vi "Process.vi"(8 "error in":errorcluster, 11 "Qbus in":refnum<class "Qbus.lvclass">) -> (0 "error out":errorcluster)   [LabVIEW 2021, in "DigitalAudioGenerationProcess.lvlib"]
uses:
  DigitalAudioGenerationProcess.lvlib
  <vilib>/addons/Qbus/Qbus.lvclass
  controls/state.ctl
  controls/generation status.ctl
  <vilib>/PDM Acquisition Toolkit/host/Classes/Tasks/PCM Output/Controls/PCM Output Task DVR.ctl
  <vilib>/PDM Acquisition Toolkit/host/Classes/Tasks/PCM Output/PCM Output Task.lvclass
  controls/digital generation settings.ctl
  controls/digital protocol settings.ctl
  <vilib>/PDM Acquisition Toolkit/host/Classes/Session/Controls/Logic Levels.ctl
  <vilib>/PDM Acquisition Toolkit/shared/controls/PCM Data Format Configuration.ctl
  <vilib>/PDM Acquisition Toolkit/shared/controls/Digital Edge.ctl
  <vilib>/PDM Acquisition Toolkit/shared/controls/PCM Bit Endianness.ctl
  <vilib>/PDM Acquisition Toolkit/shared/controls/PCM Data Justification.ctl
  <vilib>/PDM Acquisition Toolkit/shared/controls/clock mode.ctl
  <vilib>/PDM Acquisition Toolkit/shared/controls/PCM Frame Sync Control.ctl
  <vilib>/PDM Acquisition Toolkit/host/Classes/Tasks/I2S Output/Control/SignalProperties.ctl
  <vilib>/PDM Acquisition Toolkit/host/Classes/Channels/I2S Ouput/Controls/GenerationChannelProperties.ctl
  controls/update signal settings.ctl
  <vilib>/PDM Acquisition Toolkit/host/Classes/Session/DecoderSession.lvclass
  <vilib>/PDM Acquisition Toolkit/shared/PDM Shared.lvlib
  controls/AudioGenTypeDefs.lvlib
  <vilib>/PDM Acquisition Toolkit/host/Classes/Channels/I2S Ouput/I2S Output Channel.lvclass
  <vilib>/PDM Acquisition Toolkit/host/Classes/Tasks/I2S Output/I2S Output Task.lvclass
  shared/logger process/EventLoggerProcess.lvlib
  subVIs/utility/AudioGenUtility.lvlib
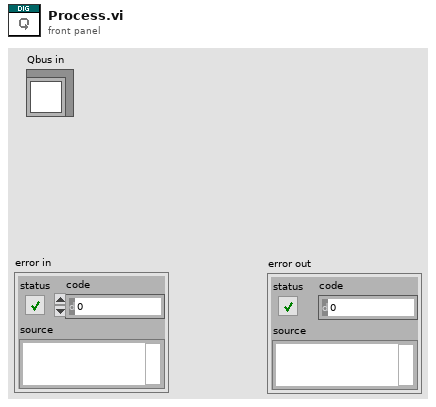
[diagram p1: front panel]
types:
  T1 = typedef "DigitalAudioGenerationProcess.lvlib/state.ctl" = cluster{"status":T2, "data task":T3, "master clock task":T3}
  T2 = typedef "AudioGenTypeDefs.lvlib/generation status.ctl" = enum16{"Idle", "Committed", "Active"}
  T3 = typedef "PDM Acquisition Class Library.lvlib/PCM Output Task.lvclass/PCM Output Task DVR.ctl" = refnum<data-value>
  T4 = typedef "AudioGenTypeDefs.lvlib/digital generation settings.ctl" = cluster{"data channel list":string, "master clock channel list":string, "digital protocol settings":T5, "signal parameters":T13}
  T5 = typedef "AudioGenTypeDefs.lvlib/digital protocol settings.ctl" = cluster{"logic level":T6, "PCM Data Configuration":T7, "bit clock rate":sgl, "master clock rate":sgl, "clock mode":T11, "Frame Sync Clock Control":T12}
  T6 = typedef "PDM Acquisition Class Library.lvlib/DecoderSession.lvclass/Logic Levels.ctl" = enum16{"3.3 V", "1.8 V", "1.2 V"}
  T7 = typedef "PDM Shared.lvlib/PCM Data Format Configuration.ctl" = cluster{"Frame Sync Edge for Channel 0":T8, "Channel Count Per Frame":u8, "Channel Length":u16, "Bit Depth":u8, "Channel 0 Offset":u16, "Endianness":T9, "Data Justification":T10}
  T8 = typedef "PDM Shared.lvlib/Digital Edge.ctl" = enum8{"Rising", "Falling"}
  T9 = typedef "PDM Shared.lvlib/PCM Bit Endianness.ctl" = enum16{"MSB First", "LSB First"}
  T10 = typedef "PDM Shared.lvlib/PCM Data Justification.ctl" = enum16{"Left Justified", "Right Justified"}
  T11 = typedef "PDM Shared.lvlib/clock mode.ctl" = enum16{"divided clock", "DDS"}
  T12 = typedef "PDM Shared.lvlib/PCM Frame Sync Control.ctl" = cluster{"Frame Length":u16, "Frame Sync Pulse Width":u16, "Bit Clock Edge  Sync":T8}
  T13 = typedef "PDM Acquisition Class Library.lvlib/I2S Output Task.lvclass/SignalProperties.ctl" = cluster{"cyclic signal":dbl[], "channel parameters":T14[]}
  T14 = typedef "PDM Acquisition Class Library.lvlib/I2S Output Channel.lvclass/GenerationChannelProperties.ctl" = cluster{"cyclic period":dbl, "cyclic phase offset":dbl, "gain":dbl}
  T15 = typedef "AudioGenTypeDefs.lvlib/update signal settings.ctl" = cluster{"frequency":dbl, "gain":dbl}
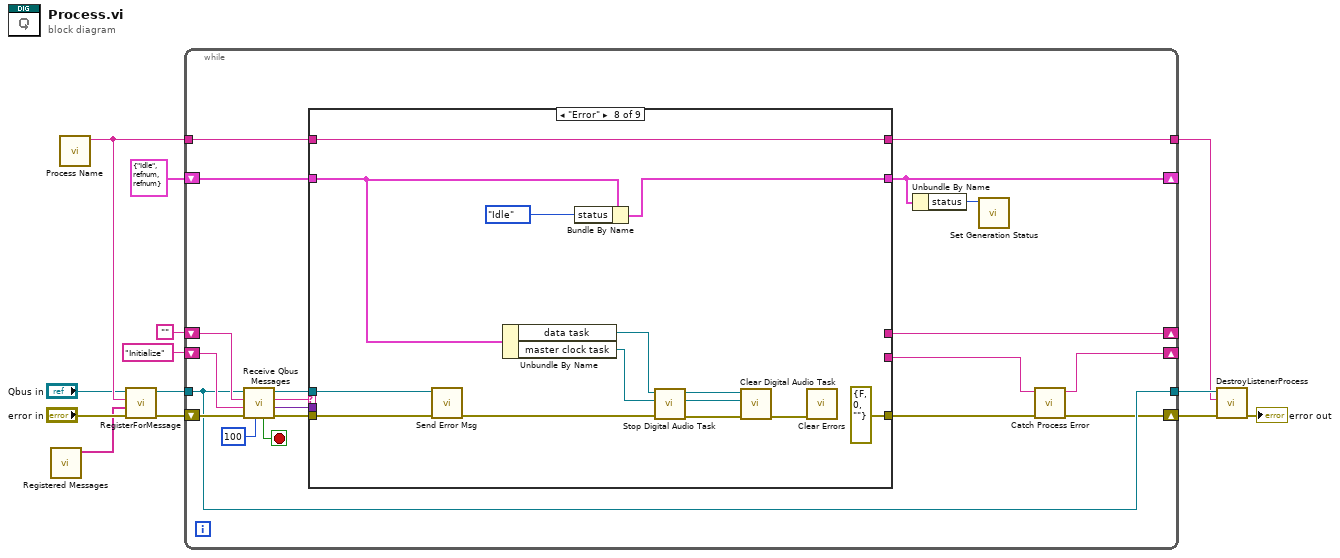
[diagram p0: block diagram]
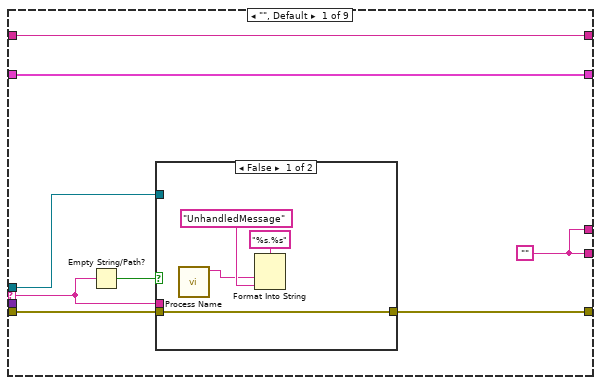
[diagram p2: hidden frame]
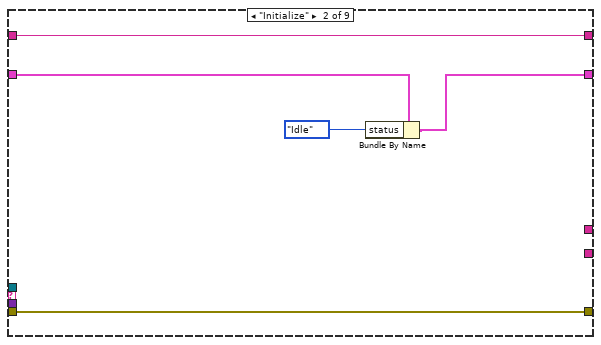
[diagram p4: hidden frame]
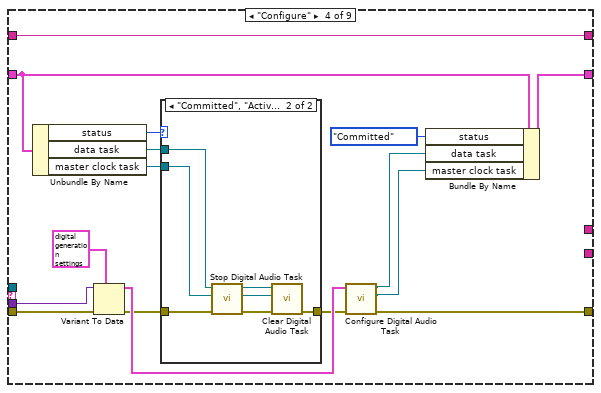
[diagram p6: hidden frame]
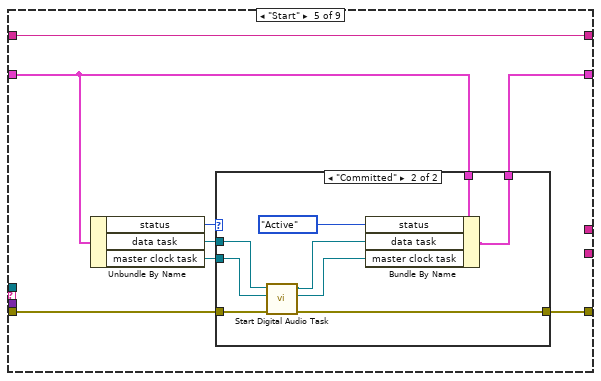
[diagram p8: hidden frame]
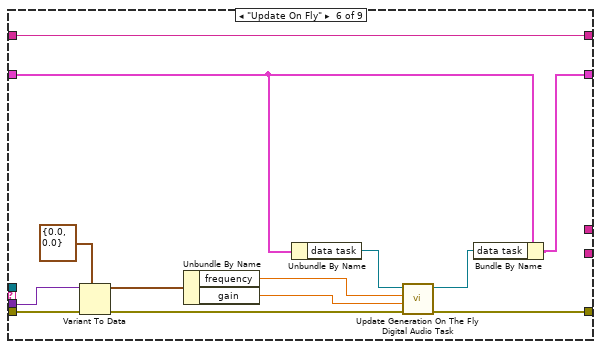
[diagram p10: hidden frame]
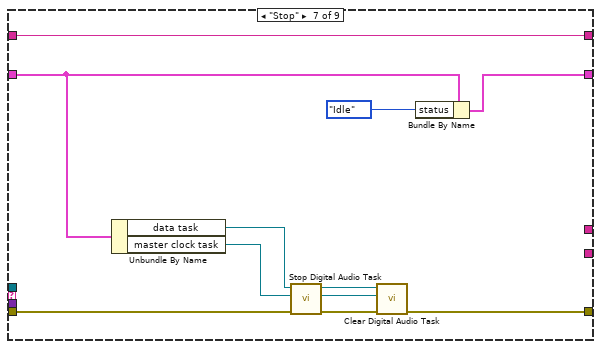
[diagram p11: hidden frame]
diagram:
  n1 = call "Registered Messages.vi"() -> ("registered messages"=w6:string[])  [unwired: 11 in]
  n2 = call "Process Name.vi"() -> ("process name"=w9:string)  [unwired: 11 in]
  n3 = call <vilib>:"RegisterForMessage.vi"("error in (no error)"="error in", "message names"=w6, "process name"=w9, "Qbus in"="Qbus in") -> ("error in (no error)"=w12:errorcluster, "Qbus out"=w13:refnum<class "Qbus.lvclass">)  [unwired: 6 in]
  n4 = while {
    shift-right: [w23] -> _
    shift-left: "" -> [w32]
    tunnel: w13 -> [w18]
    tunnel: w9 -> [w22]
    tunnel: [w18] -> w4
    tunnel: [w24] -> w2
    shift-right: [w14] -> _
    shift-left: "Initialize" -> [w28]
    shift-right: [w17] -> w5
    shift-left: w12 -> [w27]
    shift-right: [w19] -> _
    shift-left: T1 {"status"=enum."Idle", "data task"=refnum, "master clock task"=refnum} ("state") -> [w21]
    stop <- w33 stop-if-true
    n5 = call "Receive Qbus Messages.vi"("timeout(ms)"=100 ("milliseconds to wait"), "error in (no error)"=w27, "priority action"=w28, "default action"=w32, "Qbus in"=w18) -> ("error out"=w31:errorcluster, "message value"=w29:variant, "action"=w26:string, "Qbus out"=w30:refnum<class "Qbus.lvclass">, "exit"=w33:bool)  [unwired: 2 in]
    n6 = case shown="\"Error\"" w26 {
      selector: w26 -> [w38 _ _ _ _ _ _ _ _]
      tunnel: w31 -> [w40 w51 w54 w69 w85 w104 w117 w124 w138]
      tunnel: w30 -> [w36 _ _ _ _ _ _ w125 _]
      tunnel: [w39 w51 w54 w66 w80 w109 w111 errorcluster {"status"=FALSE, "code"=0, "source"=""} ("error out") w138] -> w16
      tunnel: w29 -> [_ _ _ w68 _ w103 _ _ _]
      tunnel: [w41 w50 w53 w70 w86 w110 w121 w135 w137] -> w24
      tunnel: w22 -> [w41 w50 w53 w70 w86 w110 w121 w135 w137]
      tunnel: [w35 _ _ _ _ _ _ _ _] -> w15
      tunnel: [w35 _ _ _ _ _ _ _ _] -> w23
      tunnel: w21 -> [w34 w49 w52 w60 w82 w106 w119 w133 w136]
      tunnel: [w34 w48 w52 w64 w81 w105 w118 w132 w136] -> w19
      frame "", Default {
        w35 = ""
        n7 = Empty String/Path?(string/path=w38) -> (empty?=w37:bool)
        n8 = case shown="False" w37 {
          tunnel: [w42 w46] -> w39
          tunnel: w40 -> [w42 w46]
          tunnel: w38 -> [_ _]
          tunnel: w36 -> [_ _]
          frame False {
            n9 = call "Process Name.vi"() -> ("process name"=w43:string)  [unwired: 11 in]
            n10 = Format Into String(format string="%s.%s", w43, "UnhandledMessage" ("ProcessName")) -> ()  [unwired: 2 in, 2 out]
          }
          frame True {
          }
        }
      }
      frame "Initialize" {
        n11 = Bundle By Name(cluster=w49, "status"=generation_status."Idle") -> (w48:T1)
      }
      frame "DetectHW" {
      }
      frame "Configure" {
        n12 = Unbundle By Name(w60) -> ("status"=w59:T2, "data task"=w58:T3, "master clock task"=w57:T3)
        n13 = Variant To Data(error in=w69, type=T4 {"data channel list"="", "master clock channel list"="", "digital protocol settings"={"logic level"=enum."3.3 V", "PCM Data Configuration"={"Frame Sync Edge for Channel 0"=enum."Falling", "Channel Count Per Frame"=2, "Channel Length"=32, "Bit Depth"=24, "Channel 0 Offset"=1, "Endianness"=enum."MSB First", "Data Justification"=enum."Left Justified"}, "bit clock rate"=3025000.0, "master clock rate"=3025000.0, "clock mode"=enum."divided clock", "Frame Sync Clock Control"={"Frame Length"=64, "Frame Sync Pulse Width"=32, "Bit Clock Edge  Sync"=enum."Falling"}}, "signal parameters"={"cyclic signal"=[], "channel parameters"=[]}} ("digital generation"), Variant=w68) -> (data=w65:T4, error out=w56:errorcluster)
        n14 = case shown="\"Committed\", \"Active\"" w59 {
          tunnel: w58 -> [_ w73]
          tunnel: w57 -> [_ w72]
          tunnel: w56 -> [w71 w75]
          tunnel: [w71 w74] -> w55
          frame "Idle", Default {
          }
          frame "Committed", "Active" {
            n15 = call "Stop Digital Audio Task.vi"("error in (no error)"=w75, "master clock task"=w72, "data task"=w73) -> ("error out"=w76:errorcluster, "master clock task"=w78:T3, "data task"=w77:T3)  [unwired: 6 in]
            n16 = call "Clear Digital Audio Task.vi"("error in (no error)"=w76, "master clock task"=w78, "data task"=w77) -> ("error out"=w74:errorcluster)  [unwired: 8 in]
          }
        }
        n17 = call "Configure Digital Audio Task.vi"("error in (no error)"=w55, "digital generation"=w65) -> ("error out"=w66:errorcluster, "master clock task"=w61:T3, "data task"=w62:T3)  [unwired: 7 in]
        n18 = Bundle By Name(cluster=w60, "status"=generation_status."Committed", "data task"=w62, "master clock task"=w61) -> (w64:T1)
      }
      frame "Start" {
        n19 = Unbundle By Name(w82) -> ("status"=w79:T2, "data task"=w84:T3, "master clock task"=w83:T3)
        n20 = case shown="\"Committed\"" w79 {
          tunnel: w85 -> [w88 w97]
          tunnel: w84 -> [_ w96]
          tunnel: w83 -> [_ w95]
          tunnel: w82 -> [w87 w92]
          tunnel: [w87 w91] -> w81
          tunnel: [w88 w90] -> w80
          frame "Idle", Default {
            # "not ready to start; commit first"
          }
          frame "Committed" {
            n21 = call "Start Digital Audio Task.vi"("error in (no error)"=w97, "master clock task"=w95, "data task"=w96) -> ("error out"=w90:errorcluster, "master clock task"=w93:T3, "data task"=w94:T3)  [unwired: 6 in]
            n22 = Bundle By Name(cluster=w92, "status"=generation_status."Active", "data task"=w94, "master clock task"=w93) -> (w91:T1)
          }
        }
      }
      frame "Update On Fly" {
        n23 = Variant To Data(error in=w104, type=T15 {"frequency"=0.0, "gain"=0.0} ("signal update setting"), Variant=w103) -> (data=w101:T15, error out=w100:errorcluster)
        n24 = Unbundle By Name(w101) -> ("frequency"=w99:dbl, "gain"=w98:dbl)
        n25 = Unbundle By Name(w106) -> ("data task"=w107:T3)
        n26 = call "Update Generation On The Fly Digital Audio Task.vi"("error in (no error)"=w100, "gain"=w98, "frequency"=w99, "data task"=w107) -> ("error out"=w109:errorcluster, "data task"=w108:T3)  [unwired: 6 in]
        n27 = Bundle By Name(cluster=w106, "data task"=w108) -> (w105:T1)
      }
      frame "Stop" {
        n28 = Unbundle By Name(w119) -> ("data task"=w116:T3, "master clock task"=w115:T3)
        n29 = call "Stop Digital Audio Task.vi"("error in (no error)"=w117, "master clock task"=w115, "data task"=w116) -> ("error out"=w114:errorcluster, "master clock task"=w112:T3, "data task"=w113:T3)  [unwired: 6 in]
        n30 = call "Clear Digital Audio Task.vi"("error in (no error)"=w114, "master clock task"=w112, "data task"=w113) -> ("error out"=w111:errorcluster)  [unwired: 8 in]
        n31 = Bundle By Name(cluster=w119, "status"=generation_status."Idle") -> (w118:T1)
      }
      frame "Error" {
        n32 = call "Send Error Msg.vi"("error in"=w124, "Qbus in"=w125) -> ("error out"=w123:errorcluster)  [unwired: 8 in, 1 out]
        n33 = Unbundle By Name(w133) -> ("data task"=w131:T3, "master clock task"=w130:T3)
        n34 = Bundle By Name(cluster=w133, "status"=generation_status."Idle") -> (w132:T1)
        n35 = call "Stop Digital Audio Task.vi"("error in (no error)"=w123, "master clock task"=w130, "data task"=w131) -> ("error out"=w129:errorcluster, "master clock task"=w127:T3, "data task"=w128:T3)  [unwired: 6 in]
        n36 = call "Clear Digital Audio Task.vi"("error in (no error)"=w129, "master clock task"=w127, "data task"=w128) -> ("error out"=w122:errorcluster)  [unwired: 8 in]
        n37 = call <vilib>:"Clear Errors.vi"("error in (no error)"=w122) -> ()  [unwired: 5 in, 2 out]
      }
      frame "Exit" {
      }
    }
    n38 = Unbundle By Name(w19) -> ("status"=w20:T2)
    n39 = call "Set Generation Status.vi"("status"=w20) -> ()  [unwired: 10 in, 1 out]
    n40 = call "Catch Process Error.vi"("error in (no error)"=w16, "priority action"=w15) -> ("error out"=w17:errorcluster, "priority action"=w14:string)  [unwired: 8 in]
  }
  n41 = call <vilib>:"DestroyListenerProcess.vi"("error in (no error)"=w5, "process name"=w2, "Qbus in"=w4) -> ("error in (no error)"=→"error out":errorcluster)  [unwired: 7 in, 1 out]
